vi "DrawCircle.vi"(10 "r":dbl, 11 "Center":cluster{"x":dbl, "y":dbl} {"y" scale=-10.0..10.0; "x" scale=-10.0..10.0}) -> (3 "Circle Graph":cluster{dbl, dbl}[](array[cluster]))   [LabVIEW 2018]
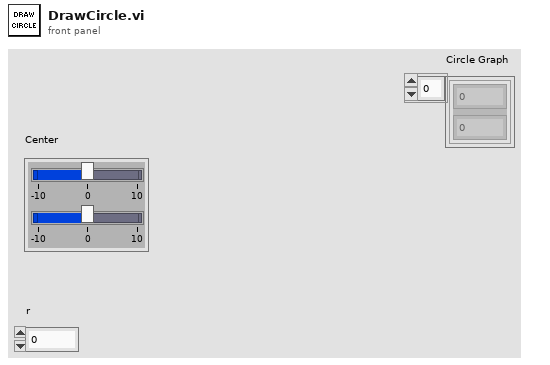
[diagram p1: front panel]
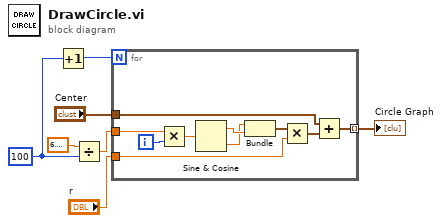
[diagram p0: block diagram]
diagram:
  w1 = 100
  n1 = Increment(x=w1) -> (x+1=w2:i32)
  n2 = Divide(x=6.283185307179586, y=w1) -> (x/y=w5:dbl)
  n3 = for {
    N: w2 -> [_]
    tunnel: "Center" -> [w10]
    tunnel: w5 -> [w17]
    tunnel: "r" -> [w11]
    tunnel: [w8] -> w3 mode=indexing
    i -> [w16]
    n4 = Multiply(x=w17, y=w16) -> (x*y=w15:dbl)
    n5 = Sine & Cosine(0:w15) -> (1:w14:dbl, 2:w13:dbl)
    n6 = Bundle(w13, w14) -> (w12:cluster{dbl, dbl})  [unwired: 1 in]
    n7 = Multiply(x=w12, y=w11) -> (x*y=w9:cluster{dbl, dbl})
    n8 = Add(x=w10, y=w9) -> (x+y=w8:cluster{dbl, dbl})
  }
  "Circle Graph" <- w3
